vi "RfSwitch_WAM_ATE.vi"(0 "VISA_IN":refnum<visa-resource-name>="GPIB0::29::INSTR", 11 "error in":errorcluster, 12 "Source":enum16{"RFSM", "PNA"}(ring), 14 "T/R":enum16{"TX", "RX"}(ring)) -> (4 "visa_out":refnum<visa-resource-name>, 15 "error out":errorcluster)   [LabVIEW 2018]
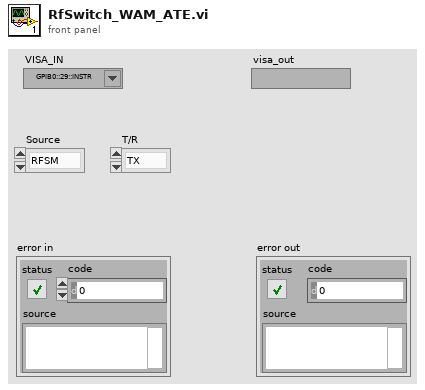
[diagram p1: front panel]
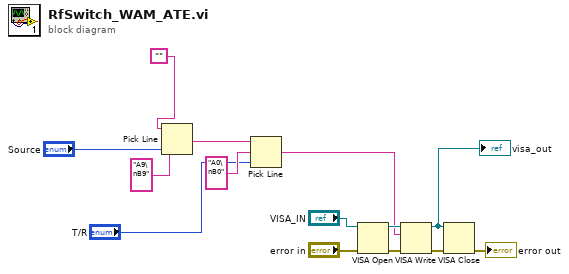
[diagram p0: block diagram]
diagram:
  n1 = Pick Line(string ("")="", multi-line string="A9\nB9", line index="Source") -> (output string=w4:string)
  n2 = Pick Line(string ("")=w4, multi-line string="A0\nB0", line index="T/R") -> (output string=w2:string)
  n3 = VISA Open(error in (no error)="error in", VISA resource name="VISA_IN") -> (VISA resource name=w13:refnum<visa-resource-name>, error out=w12:errorcluster)  [unwired: 3 in]
  n4 = VISA Write(VISA resource name=w13, write buffer=w2, error in (no error)=w12) -> (VISA resource name out=w11:refnum<visa-resource-name>, error out=w14:errorcluster)  [unwired: 1 out]
  "visa_out" <- w11
  n5 = VISA Close(VISA resource name=w11, error in (no error)=w14) -> (error out=→"error out":errorcluster)
